vi "DC_input.vi"(0 "input":T2) -> (1 "output":T1, 2 "tick":bool)   [LabVIEW 2013]
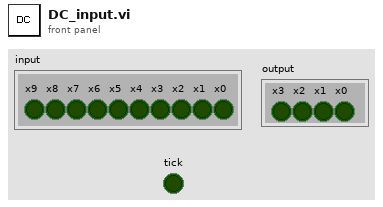
[diagram p1: front panel]
types:
  T1 = cluster{"x3":bool, "x2":bool, "x1":bool, "x0":bool}
  T2 = cluster{"x9":bool, "x8":bool, "x7":bool, "x6":bool, "x5":bool, "x4":bool, "x3":bool, "x2":bool, "x1":bool, "x0":bool}
  T3 = cluster{"x1":bool, "x2":bool, "x3":bool, "x4":bool, "x5":bool, "x6":bool, "x7":bool, "x8":bool, "x9":bool, "x0":bool}
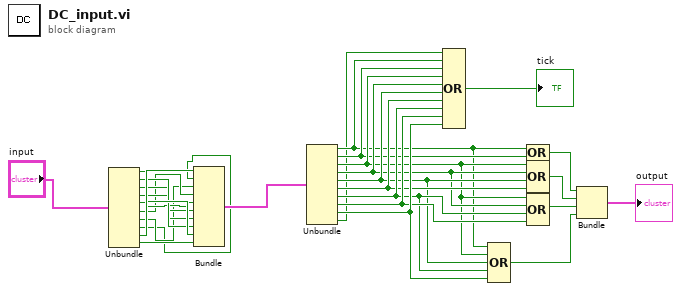
[diagram p0: block diagram]
diagram:
  n1 = Unbundle("input") -> ("x9"=w8:bool, "x8"=w7:bool, "x7"=w6:bool, "x6"=w5:bool, "x5"=w4:bool, "x4"=w3:bool, "x3"=w2:bool, "x2"=w1:bool, "x1"=w9:bool, "x0"=w10:bool)
  n2 = Bundle("x1"=w9, "x2"=w1, "x3"=w2, "x4"=w3, "x5"=w4, "x6"=w5, "x7"=w6, "x8"=w7, "x9"=w8, "x0"=w10) -> (w11:T3)  [unwired: 1 in]
  n3 = Unbundle(w11) -> ("x1"=w15:bool, "x2"=w16:bool, "x3"=w17:bool, "x4"=w18:bool, "x5"=w19:bool, "x6"=w20:bool, "x7"=w21:bool, "x8"=w22:bool, "x9"=w23:bool, "x0"=w14:bool)
  n4 = Compound Arithmetic op=OR(w14, w15, w16, w17, w18, w19, w20, w21, w22, w23) -> (→"tick":bool)
  n5 = Compound Arithmetic op=OR(w15, w17, w19, w21, w23) -> (w24:bool)
  n6 = Compound Arithmetic op=OR(w15, w16) -> (w27:bool)
  n7 = Compound Arithmetic op=OR(w17, w18, w19, w20) -> (w26:bool)
  n8 = Compound Arithmetic op=OR(w17, w18, w21, w22) -> (w25:bool)
  n9 = Bundle(w27, w26, w25, w24) -> (→"output":cluster{bool, bool, bool, bool})  [unwired: 1 in]
